vi "读取产品参数信息-孔径参数.vi"(8 "错误输入（无错误）":errorcluster, 11 "LoadProductName":string) -> (0 "错误输出":errorcluster)   [LabVIEW 2017]
uses:
  Global System.vi
panel:
  out "连接的字符串":string
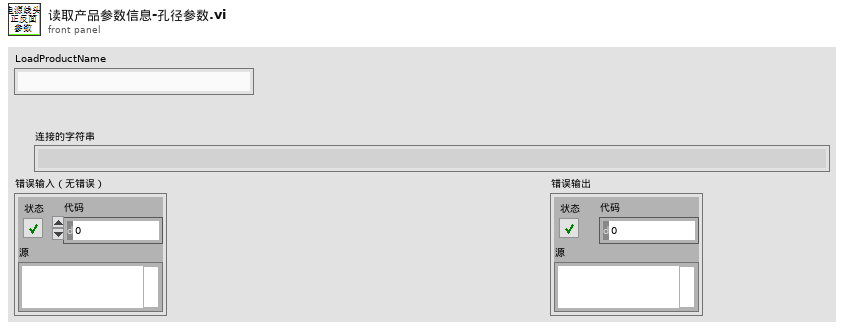
[diagram p1: front panel]
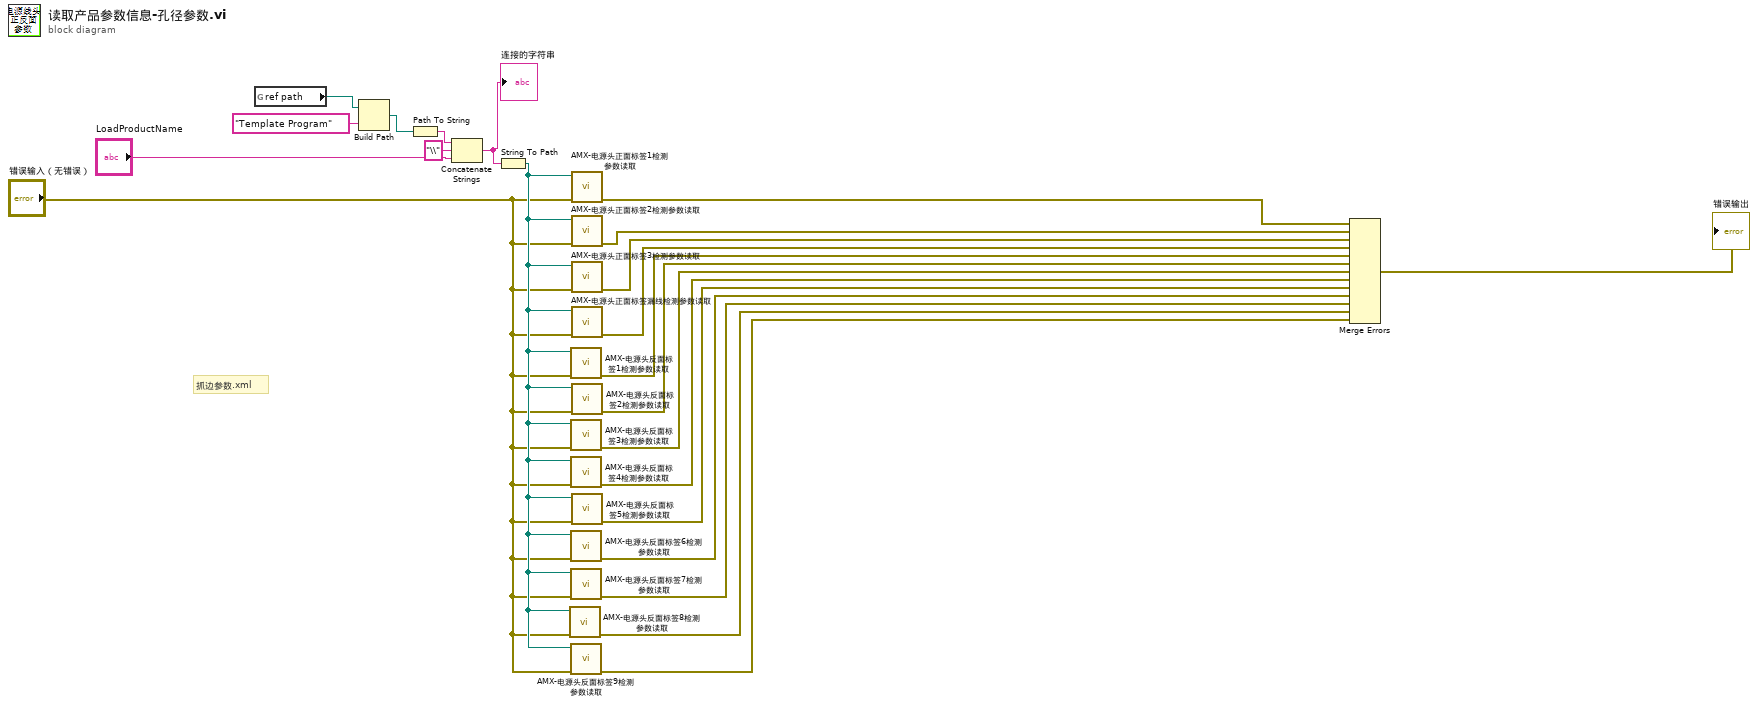
[diagram p0: block diagram]
diagram:
  # "抓边参数.xml"
  n1 = global read "Global System.vi" "ref path"() -> (w23:path)
  n2 = Build Path(base path=w23, name or relative path="Template Program" ("名称或相对路径")) -> (appended path=w21:path)
  n3 = Path To String(path=w21) -> (string=w20:string)
  n4 = Concatenate Strings(w20, "\\" ("字符串"), "LoadProductName") -> (w17:string)
  "连接的字符串" <- w17
  n5 = String To Path(string=w17) -> (path=w3:path)
  n6 = call "AMX-电源头反面标签8检测参数读取.vi"("error in (no error)"="错误输入（无错误）", "基路径"=w3) -> ("error out"=w4:errorcluster)  [unwired: 6 in, 2 out]
  n7 = call "AMX-电源头反面标签1检测参数读取.vi"("error in (no error)"="错误输入（无错误）", "基路径"=w3) -> ("error out"=w11:errorcluster)  [unwired: 6 in, 2 out]
  n8 = call "AMX-电源头反面标签3检测参数读取.vi"("error in (no error)"="错误输入（无错误）", "基路径"=w3) -> ("error out"=w9:errorcluster)  [unwired: 6 in, 2 out]
  n9 = call "AMX-电源头反面标签4检测参数读取.vi"("error in (no error)"="错误输入（无错误）", "基路径"=w3) -> ("error out"=w8:errorcluster)  [unwired: 6 in, 2 out]
  n10 = call "AMX-电源头反面标签6检测参数读取.vi"("error in (no error)"="错误输入（无错误）", "基路径"=w3) -> ("error out"=w6:errorcluster)  [unwired: 6 in, 2 out]
  n11 = call "AMX-电源头反面标签7检测参数读取.vi"("error in (no error)"="错误输入（无错误）", "基路径"=w3) -> ("error out"=w5:errorcluster)  [unwired: 6 in, 2 out]
  n12 = call "AMX-电源头反面标签9检测参数读取.vi"("error in (no error)"="错误输入（无错误）", "基路径"=w3) -> ("error out"=w1:errorcluster)  [unwired: 6 in, 2 out]
  n13 = call "AMX-电源头正面标签1检测参数读取.vi"("error in (no error)"="错误输入（无错误）", "基路径"=w3) -> ("error out"=w16:errorcluster)  [unwired: 6 in, 2 out]
  n14 = call "AMX-电源头正面标签2检测参数读取.vi"("error in (no error)"="错误输入（无错误）", "基路径"=w3) -> ("error out"=w14:errorcluster)  [unwired: 6 in, 2 out]
  n15 = call "AMX-电源头正面标签3检测参数读取.vi"("error in (no error)"="错误输入（无错误）", "基路径"=w3) -> ("error out"=w13:errorcluster)  [unwired: 6 in, 2 out]
  n16 = call "AMX-电源头正面标签漏线检测参数读取.vi"("error in (no error)"="错误输入（无错误）", "基路径"=w3) -> ("error out"=w12:errorcluster)  [unwired: 6 in, 2 out]
  n17 = call "AMX-电源头反面标签2检测参数读取.vi"("error in (no error)"="错误输入（无错误）", "基路径"=w3) -> ("error out"=w10:errorcluster)  [unwired: 6 in, 2 out]
  n18 = call "AMX-电源头反面标签5检测参数读取.vi"("error in (no error)"="错误输入（无错误）", "基路径"=w3) -> ("error out"=w7:errorcluster)  [unwired: 6 in, 2 out]
  n19 = Merge Errors(w16, w14, w13, w12, w11, w10, w9, w8, w7, w6, w5, w4, w1) -> (→"错误输出":errorcluster)
